vi "Generate PV Names.vi"(8 "error in (no error)":errorcluster) -> (0 "error out":errorcluster, 3 "map":map{string, T1}(c390))   [LabVIEW 2020]
uses:
  Value/Type Code.ctl
  <vilib>/regexp/Match Regular Expression.xnode
  Value/Value.lvlib
  <userlib>/_OpenG.lib/lvdata/lvdata.llb/openg_variant.lvlib
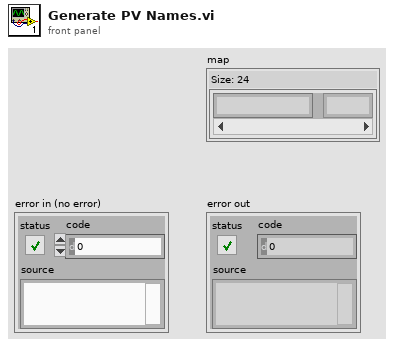
[diagram p1: front panel]
types:
  T1 = typedef "Value.lvlib/Type Code.ctl" = enum8{"Null", "Bool", "BoolA", "Int8", "Int8A", "Int16", "Int16A", "Int32", "Int32A", "Int64", "Int64A", "UInt8", "UInt8A", "UInt16", "UInt16A", "UInt32", "UInt32A", "UInt64", "UInt64A", "Float32", "Float32A", "Float64", "Float64A", "String", "StringA", "Struct", "StructA", "Union", "UnionA", "Any", "AnyA"}
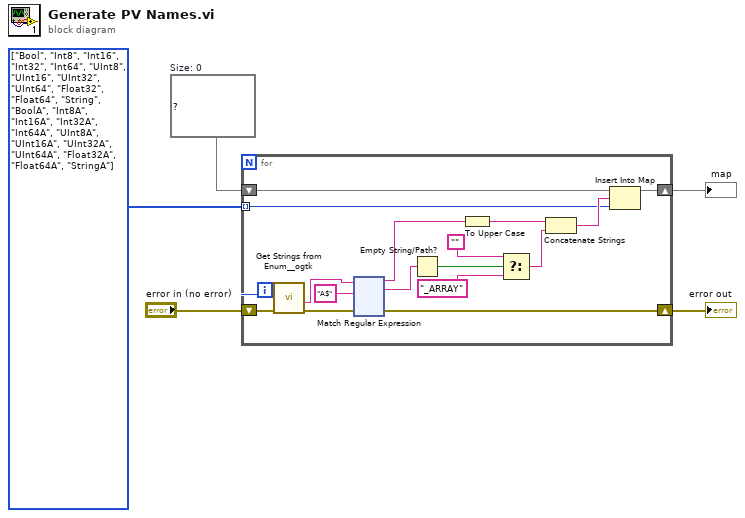
[diagram p0: block diagram]
diagram:
  w1 = T1[] [enum."Bool", enum."Int8", enum."Int16", enum."Int32", enum."Int64", enum."UInt8", enum."UInt16", enum."UInt32", enum."UInt64", enum."Float32", enum."Float64", enum."String", enum."BoolA", enum."Int8A", enum."Int16A", enum."Int32A", enum."Int64A", enum."UInt8A", enum."UInt16A", enum."UInt32A", enum."UInt64A", enum."Float32A", enum."Float64A", enum."StringA"] items=["Null", "Bool", "BoolA", "Int8", "Int8A", "Int16", "Int16A", "Int32", "Int32A", "Int64", "Int64A", "UInt8", "UInt8A", "UInt16", "UInt16A", "UInt32", "UInt32A", "UInt64", "UInt64A", "Float32", "Float32A", "Float64", "Float64A", "String", "StringA", "Struct", "StructA", "Union", "UnionA", "Any", "AnyA"]
  w5 = map{string, T1} {}  # Size: 0
  n1 = for {
    tunnel: w1 -> [w7] mode=indexing
    shift-right: [w20] -> w3
    shift-left: "error in (no error)" -> [w8]
    shift-right: [w13] -> w4
    shift-left: w5 -> [w14]
    n2 = call <userlib>:"Get Strings from Enum__ogtk.vi"("error in (no error)"=w8, "Enum"=w7) -> ("error out"=w9:errorcluster, "String Value"=w6:string)  [unwired: 6 in, 2 out]
    n3 = xnode "Match Regular Expression"("input string"=w6, "regular expression"="A$", "error in"=w9) -> ("before match"=w10:string, "whole match"=w19:string, "error out"=w20:errorcluster)  [unwired: 3 in, 2 out]
    n4 = Empty String/Path?(string/path=w19) -> (empty?=w18:bool)
    n5 = To Upper Case(1:w10) -> (0:w11:string)
    n6 = Select(t="", s=w18, f="_ARRAY" ("regular expression")) -> (s? t:f=w16:string)
    n7 = Concatenate Strings(w11, w16) -> (w12:string)
    n8 = Insert Into Map(map in=w14, key=w12, value=w7) -> (map out=w13:map{string, T1})  [unwired: 2 out]
  }
  "map" <- w4
  "error out" <- w3
